vi "OnButton.vi"(0 "Button":bool, 1 "Mode":enum16{"Press", "Release", "Both"}(ring)) -> (2 "Value":bool)   [LabVIEW 2015]
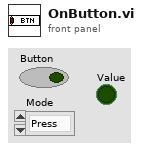
[diagram p1: front panel]
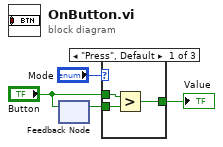
[diagram p0: block diagram]
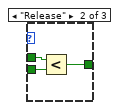
[diagram p2: hidden frame]
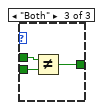
[diagram p3: hidden frame]
diagram:
  n1 = feedback-in #1("Button") -> ()
  n2 = feedback #1() -> (w3:bool)  [unwired: 1 in]
  n3 = case shown="\"Press\", Default" "Mode" {
    tunnel: w3 -> [w6 w10 w13]
    tunnel: "Button" -> [w7 w9 w12]
    tunnel: [w5 w8 w11] -> w1
    frame "Press", Default {
      n4 = Greater?(x=w7, y=w6) -> (0:w5:bool)
    }
    frame "Release" {
      n5 = Less?(x=w9, y=w10) -> (x < y?=w8:bool)
    }
    frame "Both" {
      n6 = Not Equal?(x=w12, y=w13) -> (x != y?=w11:bool)
    }
  }
  "Value" <- w1
